vi "Gait Event Detector.vi"(7 "GPD Message  In":T4) -> (1 "GPD State":T1=enum."Idle", 2 "GPD Log Msg Out":T2, 3 "Stim Msg Out":T3)   [LabVIEW 2019]
uses:
  <extravilib>/ChannelInstances/Messenger-t'GPD Message.ctl'/))Channel.ctl
  Lee Lab/CP FES Walking 2018/Code/Working/LabVIEW/Controls/Messages/GPD Message.ctl
  Lee Lab/CP FES Walking 2018/Code/Working/LabVIEW/Controls/States/GPD State.ctl
  <extravilib>/ChannelInstances/Messenger-t'Stim Message.ctl'/))Channel.ctl
  Lee Lab/CP FES Walking 2018/Code/Working/LabVIEW/Controls/Messages/Stim Message.ctl
  Lee Lab/CP FES Walking 2018/Code/Working/LabVIEW/Controls/States/Stim State.ctl
  <extravilib>/ChannelInstances/Messenger-t'Log Message.ctl'/))Channel.ctl
  Lee Lab/CP FES Walking 2018/Code/Working/LabVIEW/Controls/Messages/Log Message.ctl
  Lee Lab/CP FES Walking 2018/Code/Working/LabVIEW/Controls/States/Log State.ctl
  Controls/Event Data.ctl
  Controls/Side Event Data.ctl
  Controls/GPD Parameters.ctl
  Controls/GPD Parameter Names.ctl
  Controls/GPD Side Parameters.ctl
  Controls/Gyro Data.ctl
  Controls/Gyro Side Data.ctl
  Controls/Gyro Negation.ctl
  <extravilib>/ChannelInstances/Messenger-t'GPD Message.ctl'/Read With Abort.vi
  <extravilib>/ChannelInstances/Messenger-t'Log Message.ctl'/Write With Abort.vi
  <extravilib>/ChannelInstances/Messenger-t'Stim Message.ctl'/Write With Abort.vi
  <resource>/Channels/Messenger/Read With Abort.vi
  <vilib>/ChannelSupport/Channel Message/Read ID.vi
  <resource>/Channels/Messenger/Write With Abort.vi
  <extravilib>/ChannelInstances/Messenger-t'Log Message.ctl'/Wrapper.lvclass
  C:/Program Files/National Instruments/LabVIEW 2019/vi.lib/ChannelSupport/Channel Message/Channel Message.lvclass
  <extravilib>/ChannelInstances/Messenger-t'Stim Message.ctl'/Wrapper.lvclass
  <resource>/Channels/Messenger/Endpoint.vi
  <extravilib>/ChannelInstances/Messenger-t'GPD Message.ctl'/Unwrap.vi
  <extravilib>/ChannelInstances/Messenger-t'Log Message.ctl'/Wrap.vi
  <extravilib>/ChannelInstances/Messenger-t'Stim Message.ctl'/Wrap.vi
  <extravilib>/ChannelInstances/Messenger-t'GPD Message.ctl'.lvlib
  <extravilib>/ChannelInstances/Messenger-t'Stim Message.ctl'.lvlib
  <extravilib>/ChannelInstances/Messenger-t'Log Message.ctl'.lvlib
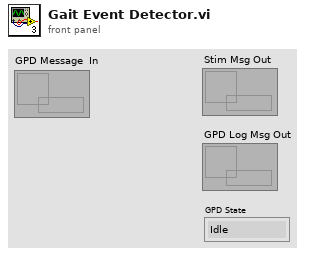
[diagram p1: front panel]
types:
  T1 = typedef "GPD State.ctl" = enum16{"On", "Stop", "Idle", "Initialize", "Update GPD Params", "Reload GPD Params", "Detect Event"}
  T2 = typedef "Messenger-t'Log Message.ctl'.lvlib/))Channel.ctl" = refnum<queue>
  T3 = typedef "Messenger-t'Stim Message.ctl'.lvlib/))Channel.ctl" = refnum<queue>
  T4 = typedef "Messenger-t'GPD Message.ctl'.lvlib/))Channel.ctl" = refnum<queue>
  T5 = typedef "GPD Message.ctl" = cluster{"GPD State":T1, "Data":variant}
  T6 = typedef "GPD Parameters.ctl" = cluster{"Parameter Name":T7, "Left":T8, "Right":T8}
  T7 = typedef "GPD Parameter Names.ctl" = string[]
  T8 = typedef "GPD Side Parameters.ctl" = cluster{"% Cycle Delay":dbl, "Min % Cycle LR to ISw ":dbl, "Min % Cycle LR to MSw":dbl, "Min % Cycle LR to TSw":dbl, "Max % Cycle ISw to MSw":dbl, "Min % Cycle TSw to LR":dbl, "Max % Cycle TSw to LR":dbl, "LR Min Gyro Z Threshold":dbl, "LR Min Gyro Z Width":dbl, "ISw Peak Threshold":dbl, "ISw Peak Width":dbl, "TSw Valley Threshold":dbl, "TSw Valley Width (ms)":dbl, "Max Cycle Time (s)":dbl, "Mean Computation Window":dbl, "CP subject?":bool}
  T9 = typedef "Event Data.ctl" = cluster{"Mean Cycle Duration":dbl, "Left Event Data":T10, "Right Event Data":T10, "Numeric":dbl}
  T10 = typedef "Side Event Data.ctl" = cluster{"Event Data":cluster{"LR":cluster{"Phase":string, "On":bool, "Last On Time":dbl, "Duration":dbl, "Crossing Time":dbl, "Time since LR":dbl, "Time Since TSw":dbl, "Min gyro Z":dbl, "Time since LR?":bool, "Time since TSw?":bool, "Min gyro Z?":bool, "Crossing?":bool}, "MSt":cluster{"Phase":string, "On":bool, "Last On Time":dbl, "Duration":dbl}, "TSt":cluster{"Phase":string, "On":bool, "Last On Time":dbl, "Duration":dbl}, "PSw":cluster{"Phase":string, "On":bool, "Last On Time":dbl, "Duration":dbl}, "ISw":cluster{"Phase":string, "On":bool, "Last On Time":dbl, "Duration":dbl, "Peak Time":dbl, "Time since LR":dbl, "Time since ISw":dbl, "Time since LR?":bool, "Time since ISw?":bool, "Peak?":bool}, "MSw":cluster{"Phase":string, "On":bool, "Last On Time":dbl, "Duration":dbl, "Crossing time":dbl, "Time since LR":dbl, "Time since MSw":dbl, "Time since ISw":dbl, "Time since LR?":bool, "Time since MSw?":bool, "Time since ISw?":bool, "Crossing?":bool}, "TSw":cluster{"Phase":string, "On":bool, "Last On Time":dbl, "Duration":dbl, "Peak time":dbl, "Time since LR":dbl, "Time since TSw":dbl, "Time since LR?":bool, "Time since TSw?":bool, "Peak?":bool}}, "Mean Cycle Duration":dbl, "Event Detected?":bool, "Last Event Detected":i32, "Num Cycles":dbl, "GPD Log":refnum<queue>, "Last Event Time":dbl}
  T11 = typedef "Gyro Data.ctl" = cluster{"Time":dbl, "Normalization Time":dbl, "Sampling Rate":dbl, "Left Gyro Data":T12, "Right Gyro Data":T12}
  T12 = typedef "Gyro Side Data.ctl" = cluster{"Time":dbl, "Gyro Array Data":dbl[], "Gyro Negation":T13, "Gyro Data":cluster{"Gyro X":dbl, "Gyro Y":dbl, "Gyro Z":dbl}, "Gyro Latency":dbl, "Normalization Time":dbl, "Sampling Rate":dbl}
  T13 = typedef "Gyro Negation.ctl" = bool[]
  T14 = typedef "Event Data for Plot and Log.ctl" = cluster{"Event Deteted?":bool, "Event Data":cluster{"Right Event Time":dbl, "Left Event Time":dbl, "Right Phase":i32, "Left Phase":i32}}
  T15 = cluster{"Right Event Time":dbl, "Left Event Time":dbl, "Right Phase":i32, "Left Phase":i32}
  T16 = typedef "Log Message.ctl" = cluster{"Log State":T17, "Data":variant}
  T17 = typedef "Log State.ctl" = enum16{"Open", "Initialize", "Update", "On", "Off", "Idle", "Close", "Quit"}
  T18 = typedef "Stim Message.ctl" = cluster{"Stim State":T19, "Data":variant}
  T19 = typedef "Stim State.ctl" = enum16{"Initialize", "Open", "Idle", "Start Stim", "Update Params", "GPD Update", "Stop Stim", "Close", "Quit", "Clear Log"}
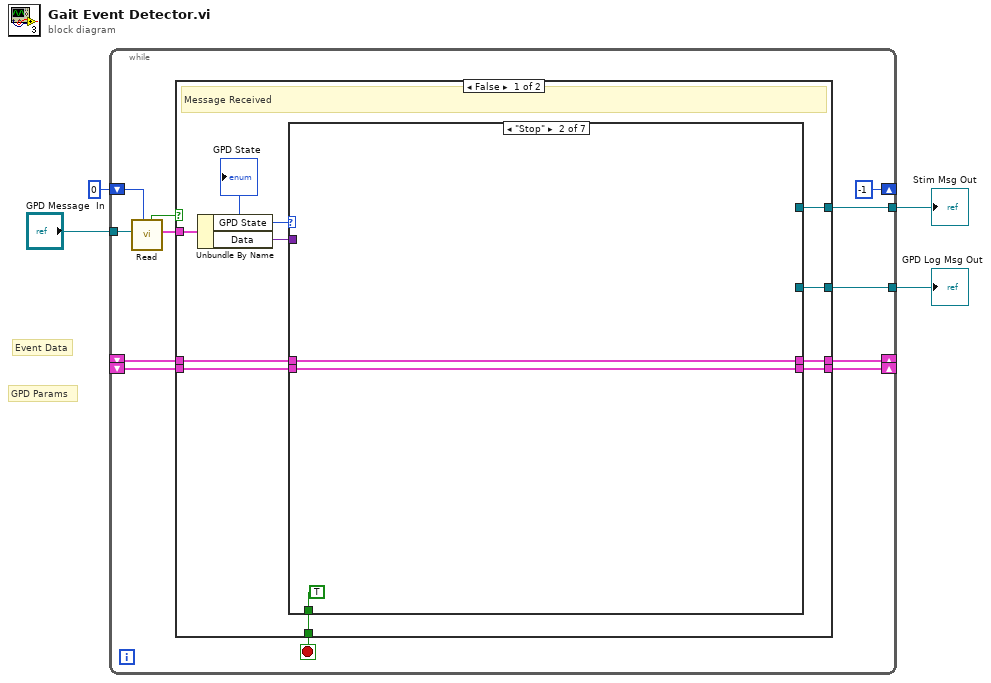
[diagram p0: block diagram]
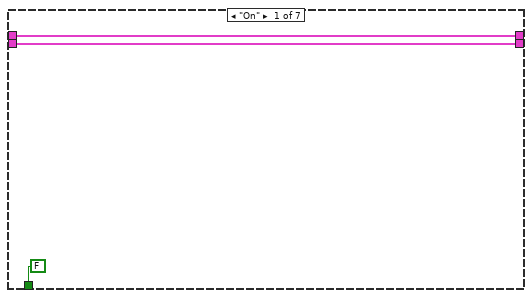
[diagram p2: hidden frame]
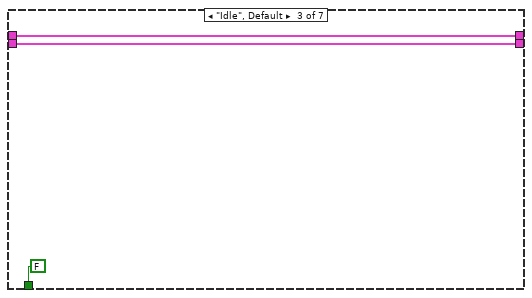
[diagram p3: hidden frame]
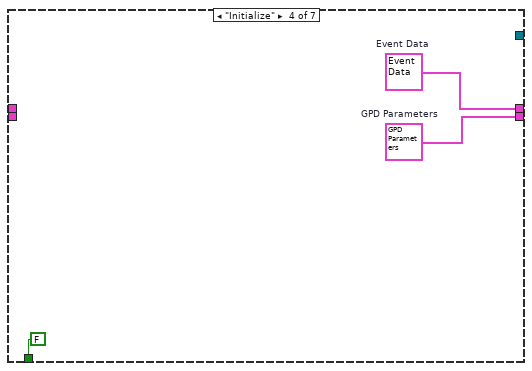
[diagram p4: hidden frame]
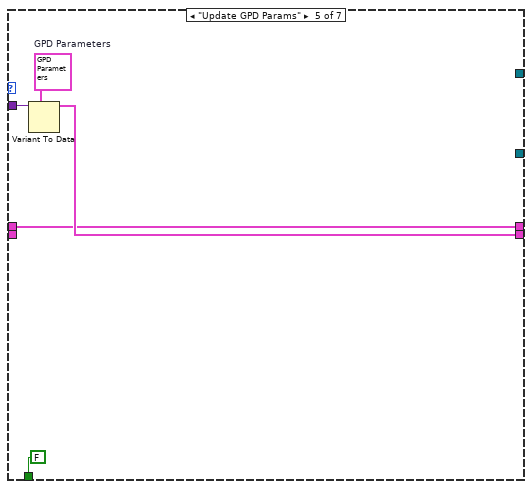
[diagram p5: hidden frame]
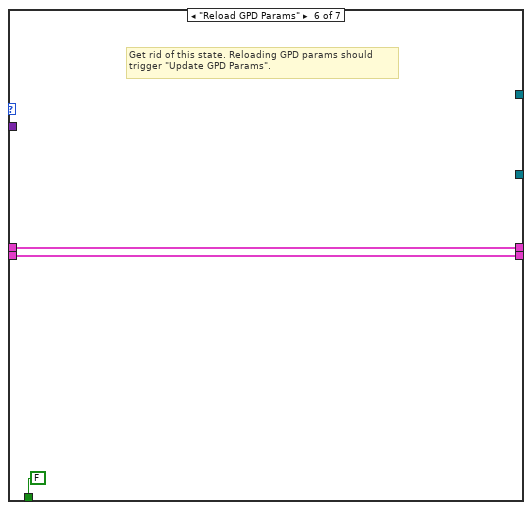
[diagram p6: hidden frame]
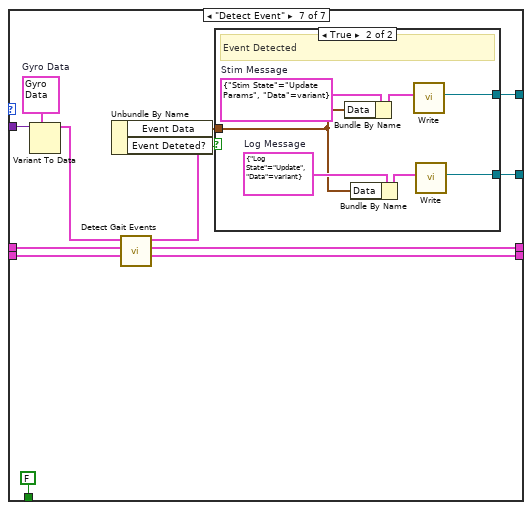
[diagram p7: hidden frame]
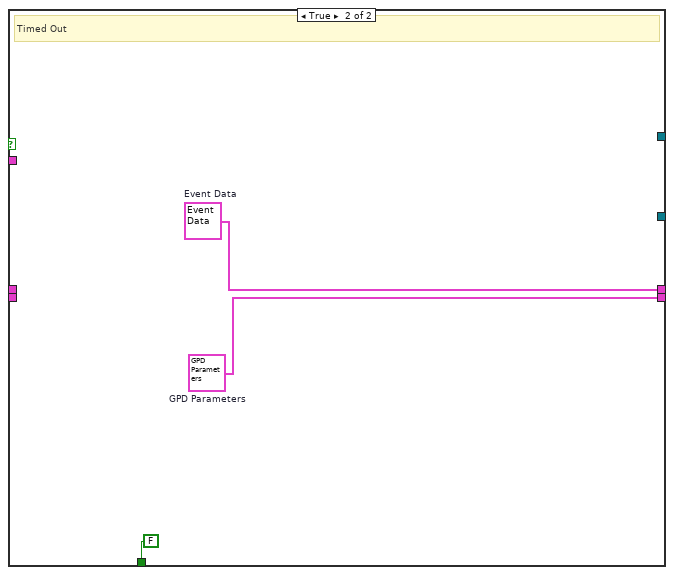
[diagram p9: hidden frame]
diagram:
  # "GPD Params"
  # "Event Data"
  n1 = while {
    tunnel: "GPD Message  In" -> [w16]
    shift-right: [w12] -> _
    shift-left: _ -> [w11]
    shift-right: [w10] -> _
    shift-left: _ -> [w9]
    tunnel: [w8] -> w3
    tunnel: [w7] -> w2
    shift-right: [-1 ("timeout in ms (-1)")] -> _
    shift-left: 0 ("timeout in ms (-1)") -> [w6]
    stop <- w13 stop-if-true
    n2 = call <extravilib>:"Read.vi"("timeout in ms (-1)"=w6, "channel"=w16) -> ("element"=w14:T5, "timedout?"=w15:bool)  [unwired: 6 in, 2 out]
    n3 = case shown="False" w15 {
      tunnel: w14 -> [w26 _]
      tunnel: [w17 FALSE] -> w13
      tunnel: w11 -> [w23 _]
      tunnel: [w22 w68] -> w12
      tunnel: [w21 w67] -> w10
      tunnel: w9 -> [w20 _]
      tunnel: [w19 _] -> w8
      tunnel: [w18 _] -> w7
      frame False {
        # "Message Received"
        n4 = Unbundle By Name(w26) -> ("GPD State"=w25:T1, "Data"=w24:variant)
        "GPD State" <- w25
        n5 = case shown="\"Stop\"" w25 {
          tunnel: w24 -> [_ _ _ _ w42 _ w59]
          tunnel: w23 -> [w28 w32 w34 _ w39 w46 w56]
          tunnel: [w28 w32 w34 w37 w39 w46 w55] -> w22
          tunnel: [w27 w31 w33 w36 w40 w45 w54] -> w21
          tunnel: w20 -> [w27 w31 w33 _ _ w45 w53]
          tunnel: [_ _ _ _ _ _ w49] -> w19
          tunnel: [_ _ _ _ _ _ w48] -> w18
          tunnel: [FALSE TRUE FALSE FALSE FALSE FALSE FALSE] -> w17
          frame "On" {
          }
          frame "Stop" {
          }
          frame "Idle", Default {
          }
          frame "Initialize" {
            w36 = T6 {"Parameter Name"=["% Cycle Delay", "Min % Cycle LR to ISw ", "Min % Cycle LR to MSw", "Min % Cycle LR to TSw", "Min % Cycle ISw to MSw", "Min % Cycle TSw to LR", "Max % Cycle TSw to LR", "LR Min Gyro Z Threshold", "LR Min Gyro Z Width", "ISw Peak Threshold", "ISw Peak Width (ms)", "TSw Valley Threshold", "TSw Valley Width (ms)", "Max Cycle Time (s)", "Mean Computation Window"], "Left"={"% Cycle Delay"=75.0, "Min % Cycle LR to ISw "=55.0, "Min % Cycle LR to MSw"=50.0, "Min % Cycle LR to TSw"=75.0, "Max % Cycle ISw to MSw"=10.0, "Min % Cycle TSw to LR"=2.5, "Max % Cycle TSw to LR"=75.0, "LR Min Gyro Z Threshold"=-0.3, "LR Min Gyro Z Width"=230.0, "ISw Peak Threshold"=0.6, "ISw Peak Width"=55.0, "TSw Valley Threshold"=-0.5, "TSw Valley Width (ms)"=55.0, "Max Cycle Time (s)"=1.3, "Mean Computation Window"=10.0, "CP subject?"=FALSE}, "Right"={"% Cycle Delay"=75.0, "Min % Cycle LR to ISw "=55.0, "Min % Cycle LR to MSw"=50.0, "Min % Cycle LR to TSw"=75.0, "Max % Cycle ISw to MSw"=10.0, "Min % Cycle TSw to LR"=2.5, "Max % Cycle TSw to LR"=75.0, "LR Min Gyro Z Threshold"=-0.3, "LR Min Gyro Z Width"=230.0, "ISw Peak Threshold"=0.6, "ISw Peak Width"=55.0, "TSw Valley Threshold"=-0.5, "TSw Valley Width (ms)"=55.0, "Max Cycle Time (s)"=1.3, "Mean Computation Window"=10.0, "CP subject?"=FALSE}}  # GPD Parameters
            w37 = T9 {"Mean Cycle Duration"=0.0, "Left Event Data"={"Event Data"={"LR"={"Phase"="LR", "On"=FALSE, "Last On Time"=0.0, "Duration"=0.0, "Crossing Time"=0.0, "Time since LR"=0.0, "Time Since TSw"=0.0, "Min gyro Z"=0.0, "Time since LR?"=FALSE, "Time since TSw?"=FALSE, "Min gyro Z?"=FALSE, "Crossing?"=FALSE}, "MSt"={"Phase"="MSt", "On"=FALSE, "Last On Time"=0.0, "Duration"=0.0}, "TSt"={"Phase"="TSt", "On"=FALSE, "Last On Time"=0.0, "Duration"=0.0}, "PSw"={"Phase"="PSw", "On"=FALSE, "Last On Time"=0.0, "Duration"=0.0}, "ISw"={"Phase"="ISw", "On"=FALSE, "Last On Time"=0.0, "Duration"=0.0, "Peak Time"=0.0, "Time since LR"=0.0, "Time since ISw"=0.0, "Time since LR?"=FALSE, "Time since ISw?"=FALSE, "Peak?"=FALSE}, "MSw"={"Phase"="MSw", "On"=FALSE, "Last On Time"=0.0, "Duration"=0.0, "Crossing time"=0.0, "Time since LR"=0.0, "Time since MSw"=0.0, "Time since ISw"=0.0, "Time since LR?"=FALSE, "Time since MSw?"=FALSE, "Time since ISw?"=FALSE, "Crossing?"=FALSE}, "TSw"={"Phase"="TSw", "On"=FALSE, "Last On Time"=0.0, "Duration"=0.0, "Peak time"=0.0, "Time since LR"=0.0, "Time since TSw"=0.0, "Time since LR?"=FALSE, "Time since TSw?"=FALSE, "Peak?"=FALSE}}, "Mean Cycle Duration"=0.0, "Event Detected?"=FALSE, "Last Event Detected"=0, "Num Cycles"=0.0, "GPD Log"=refnum, "Last Event Time"=0.0}, "Right Event Data"={"Event Data"={"LR"={"Phase"="LR", "On"=FALSE, "Last On Time"=0.0, "Duration"=0.0, "Crossing Time"=0.0, "Time since LR"=0.0, "Time Since TSw"=0.0, "Min gyro Z"=0.0, "Time since LR?"=FALSE, "Time since TSw?"=FALSE, "Min gyro Z?"=FALSE, "Crossing?"=FALSE}, "MSt"={"Phase"="MSt", "On"=FALSE, "Last On Time"=0.0, "Duration"=0.0}, "TSt"={"Phase"="TSt", "On"=FALSE, "Last On Time"=0.0, "Duration"=0.0}, "PSw"={"Phase"="PSw", "On"=FALSE, "Last On Time"=0.0, "Duration"=0.0}, "ISw"={"Phase"="ISw", "On"=FALSE, "Last On Time"=0.0, "Duration"=0.0, "Peak Time"=0.0, "Time since LR"=0.0, "Time since ISw"=0.0, "Time since LR?"=FALSE, "Time since ISw?"=FALSE, "Peak?"=FALSE}, "MSw"={"Phase"="MSw", "On"=FALSE, "Last On Time"=0.0, "Duration"=0.0, "Crossing time"=0.0, "Time since LR"=0.0, "Time since MSw"=0.0, "Time since ISw"=0.0, "Time since LR?"=FALSE, "Time since MSw?"=FALSE, "Time since ISw?"=FALSE, "Crossing?"=FALSE}, "TSw"={"Phase"="TSw", "On"=FALSE, "Last On Time"=0.0, "Duration"=0.0, "Peak time"=0.0, "Time since LR"=0.0, "Time since TSw"=0.0, "Time since LR?"=FALSE, "Time since TSw?"=FALSE, "Peak?"=FALSE}}, "Mean Cycle Duration"=0.0, "Event Detected?"=FALSE, "Last Event Detected"=0, "Num Cycles"=0.0, "GPD Log"=refnum, "Last Event Time"=0.0}, "Numeric"=0.0}  # Event Data
          }
          frame "Update GPD Params" {
            w41 = T6 {"Parameter Name"=["% Cycle Delay", "Min % Cycle LR to ISw ", "Min % Cycle LR to MSw", "Min % Cycle LR to TSw", "Min % Cycle ISw to MSw", "Min % Cycle TSw to LR", "Max % Cycle TSw to LR", "LR Min Gyro Z Threshold", "LR Min Gyro Z Width", "ISw Peak Threshold", "ISw Peak Width (ms)", "TSw Valley Threshold", "TSw Valley Width (ms)", "Max Cycle Time (s)", "Mean Computation Window"], "Left"={"% Cycle Delay"=75.0, "Min % Cycle LR to ISw "=55.0, "Min % Cycle LR to MSw"=50.0, "Min % Cycle LR to TSw"=75.0, "Max % Cycle ISw to MSw"=10.0, "Min % Cycle TSw to LR"=2.5, "Max % Cycle TSw to LR"=75.0, "LR Min Gyro Z Threshold"=-0.3, "LR Min Gyro Z Width"=230.0, "ISw Peak Threshold"=0.6, "ISw Peak Width"=55.0, "TSw Valley Threshold"=-0.5, "TSw Valley Width (ms)"=55.0, "Max Cycle Time (s)"=1.3, "Mean Computation Window"=10.0, "CP subject?"=FALSE}, "Right"={"% Cycle Delay"=75.0, "Min % Cycle LR to ISw "=55.0, "Min % Cycle LR to MSw"=50.0, "Min % Cycle LR to TSw"=75.0, "Max % Cycle ISw to MSw"=10.0, "Min % Cycle TSw to LR"=2.5, "Max % Cycle TSw to LR"=75.0, "LR Min Gyro Z Threshold"=-0.3, "LR Min Gyro Z Width"=230.0, "ISw Peak Threshold"=0.6, "ISw Peak Width"=55.0, "TSw Valley Threshold"=-0.5, "TSw Valley Width (ms)"=55.0, "Max Cycle Time (s)"=1.3, "Mean Computation Window"=10.0, "CP subject?"=FALSE}}  # GPD Parameters
            n6 = Variant To Data(type=w41, Variant=w42) -> (data=w40:T6)  [unwired: 1 in, 1 out]
          }
          frame "Reload GPD Params" {
            # "Get rid of this state. Reloading GPD params should \ntrigger \"Update GPD Params\"."
          }
          frame "Detect Event" {
            w58 = T11 {"Time"=0.0, "Normalization Time"=0.0, "Sampling Rate"=0.0, "Left Gyro Data"={"Time"=0.0, "Gyro Array Data"=[], "Gyro Negation"=[], "Gyro Data"={"Gyro X"=0.0, "Gyro Y"=0.0, "Gyro Z"=0.0}, "Gyro Latency"=0.0, "Normalization Time"=0.0, "Sampling Rate"=0.0}, "Right Gyro Data"={"Time"=0.0, "Gyro Array Data"=[], "Gyro Negation"=[], "Gyro Data"={"Gyro X"=0.0, "Gyro Y"=0.0, "Gyro Z"=0.0}, "Gyro Latency"=0.0, "Normalization Time"=0.0, "Sampling Rate"=0.0}}  # Gyro Data
            n7 = Variant To Data(type=w58, Variant=w59) -> (data=w57:T11)  [unwired: 1 in, 1 out]
            n8 = call "Detect Gait Events.vi"("GPD Parameters"=w53, "Event Data in"=w56, "Gyro Data"=w57) -> ("GPD Parameters"=w54:T6, "Event Data out"=w55:T9, "Event Data for Log and Plot"=w52:T14)  [unwired: 2 in]
            n9 = Unbundle By Name(w52) -> ("Event Data"=w50:T15, "Event Deteted?"=w51:bool)
            n10 = case shown="True" w51 {
              tunnel: w50 -> [_ w62]
              tunnel: [_ w64] -> w49
              tunnel: [_ w60] -> w48
              frame False {
                # "No Event Detected"
              }
              frame True {
                w63 = T16 {"Log State"=enum."Update", "Data"=variant}  # Log Message
                w66 = T18 {"Stim State"=enum."Update Params", "Data"=variant}  # Stim Message
                # "Event Detected"
                n11 = Bundle By Name(cluster=w66, "Data"=w62) -> (w65:T18)
                n12 = Bundle By Name(cluster=w63, "Data"=w62) -> (w61:T16)
                n13 = call <extravilib>:"Write.vi"("element"=w65) -> ("channel"=w64:T3)  [unwired: 8 in, 2 out]
                n14 = call <extravilib>:"Write.vi"("element"=w61) -> ("channel"=w60:T2)  [unwired: 8 in, 2 out]
              }
            }
          }
        }
      }
      frame True {
        w67 = T6 {"Parameter Name"=["% Cycle Delay", "Min % Cycle LR to ISw ", "Min % Cycle LR to MSw", "Min % Cycle LR to TSw", "Min % Cycle ISw to MSw", "Min % Cycle TSw to LR", "Max % Cycle TSw to LR", "LR Min Gyro Z Threshold", "LR Min Gyro Z Width", "ISw Peak Threshold", "ISw Peak Width (ms)", "TSw Valley Threshold", "TSw Valley Width (ms)", "Max Cycle Time (s)", "Mean Computation Window"], "Left"={"% Cycle Delay"=75.0, "Min % Cycle LR to ISw "=55.0, "Min % Cycle LR to MSw"=50.0, "Min % Cycle LR to TSw"=75.0, "Max % Cycle ISw to MSw"=10.0, "Min % Cycle TSw to LR"=2.5, "Max % Cycle TSw to LR"=75.0, "LR Min Gyro Z Threshold"=-0.3, "LR Min Gyro Z Width"=230.0, "ISw Peak Threshold"=0.6, "ISw Peak Width"=55.0, "TSw Valley Threshold"=-0.5, "TSw Valley Width (ms)"=55.0, "Max Cycle Time (s)"=1.3, "Mean Computation Window"=10.0, "CP subject?"=FALSE}, "Right"={"% Cycle Delay"=75.0, "Min % Cycle LR to ISw "=55.0, "Min % Cycle LR to MSw"=50.0, "Min % Cycle LR to TSw"=75.0, "Max % Cycle ISw to MSw"=10.0, "Min % Cycle TSw to LR"=2.5, "Max % Cycle TSw to LR"=75.0, "LR Min Gyro Z Threshold"=-0.3, "LR Min Gyro Z Width"=230.0, "ISw Peak Threshold"=0.6, "ISw Peak Width"=55.0, "TSw Valley Threshold"=-0.5, "TSw Valley Width (ms)"=55.0, "Max Cycle Time (s)"=1.3, "Mean Computation Window"=10.0, "CP subject?"=FALSE}}  # GPD Parameters
        w68 = T9 {"Mean Cycle Duration"=0.0, "Left Event Data"={"Event Data"={"LR"={"Phase"="LR", "On"=FALSE, "Last On Time"=0.0, "Duration"=0.0, "Crossing Time"=0.0, "Time since LR"=0.0, "Time Since TSw"=0.0, "Min gyro Z"=0.0, "Time since LR?"=FALSE, "Time since TSw?"=FALSE, "Min gyro Z?"=FALSE, "Crossing?"=FALSE}, "MSt"={"Phase"="MSt", "On"=FALSE, "Last On Time"=0.0, "Duration"=0.0}, "TSt"={"Phase"="TSt", "On"=FALSE, "Last On Time"=0.0, "Duration"=0.0}, "PSw"={"Phase"="PSw", "On"=FALSE, "Last On Time"=0.0, "Duration"=0.0}, "ISw"={"Phase"="ISw", "On"=FALSE, "Last On Time"=0.0, "Duration"=0.0, "Peak Time"=0.0, "Time since LR"=0.0, "Time since ISw"=0.0, "Time since LR?"=FALSE, "Time since ISw?"=FALSE, "Peak?"=FALSE}, "MSw"={"Phase"="MSw", "On"=FALSE, "Last On Time"=0.0, "Duration"=0.0, "Crossing time"=0.0, "Time since LR"=0.0, "Time since MSw"=0.0, "Time since ISw"=0.0, "Time since LR?"=FALSE, "Time since MSw?"=FALSE, "Time since ISw?"=FALSE, "Crossing?"=FALSE}, "TSw"={"Phase"="TSw", "On"=FALSE, "Last On Time"=0.0, "Duration"=0.0, "Peak time"=0.0, "Time since LR"=0.0, "Time since TSw"=0.0, "Time since LR?"=FALSE, "Time since TSw?"=FALSE, "Peak?"=FALSE}}, "Mean Cycle Duration"=0.0, "Event Detected?"=FALSE, "Last Event Detected"=0, "Num Cycles"=0.0, "GPD Log"=refnum, "Last Event Time"=0.0}, "Right Event Data"={"Event Data"={"LR"={"Phase"="LR", "On"=FALSE, "Last On Time"=0.0, "Duration"=0.0, "Crossing Time"=0.0, "Time since LR"=0.0, "Time Since TSw"=0.0, "Min gyro Z"=0.0, "Time since LR?"=FALSE, "Time since TSw?"=FALSE, "Min gyro Z?"=FALSE, "Crossing?"=FALSE}, "MSt"={"Phase"="MSt", "On"=FALSE, "Last On Time"=0.0, "Duration"=0.0}, "TSt"={"Phase"="TSt", "On"=FALSE, "Last On Time"=0.0, "Duration"=0.0}, "PSw"={"Phase"="PSw", "On"=FALSE, "Last On Time"=0.0, "Duration"=0.0}, "ISw"={"Phase"="ISw", "On"=FALSE, "Last On Time"=0.0, "Duration"=0.0, "Peak Time"=0.0, "Time since LR"=0.0, "Time since ISw"=0.0, "Time since LR?"=FALSE, "Time since ISw?"=FALSE, "Peak?"=FALSE}, "MSw"={"Phase"="MSw", "On"=FALSE, "Last On Time"=0.0, "Duration"=0.0, "Crossing time"=0.0, "Time since LR"=0.0, "Time since MSw"=0.0, "Time since ISw"=0.0, "Time since LR?"=FALSE, "Time since MSw?"=FALSE, "Time since ISw?"=FALSE, "Crossing?"=FALSE}, "TSw"={"Phase"="TSw", "On"=FALSE, "Last On Time"=0.0, "Duration"=0.0, "Peak time"=0.0, "Time since LR"=0.0, "Time since TSw"=0.0, "Time since LR?"=FALSE, "Time since TSw?"=FALSE, "Peak?"=FALSE}}, "Mean Cycle Duration"=0.0, "Event Detected?"=FALSE, "Last Event Detected"=0, "Num Cycles"=0.0, "GPD Log"=refnum, "Last Event Time"=0.0}, "Numeric"=0.0}  # Event Data
        # "Timed Out"
      }
    }
  }
  "Stim Msg Out" <- w3
  "GPD Log Msg Out" <- w2
